vi "gsp_simulator_write_response.vi"(4 "error in (no error)":errorcluster, 5 "Parameters":i32[](array[numeric]), 6 "Motor#":u8, 7 "Command#":u16) -> (0 "error out":errorcluster)   [LabVIEW 2015]
uses:
  gsp_simulator_global.vi
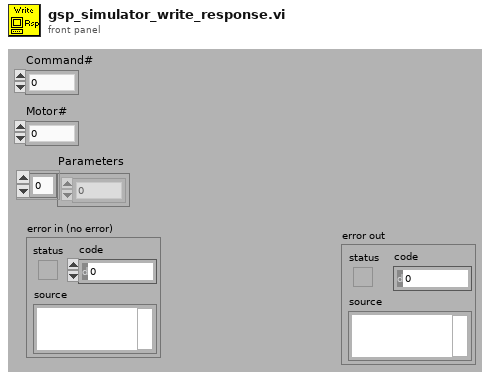
[diagram p1: front panel]
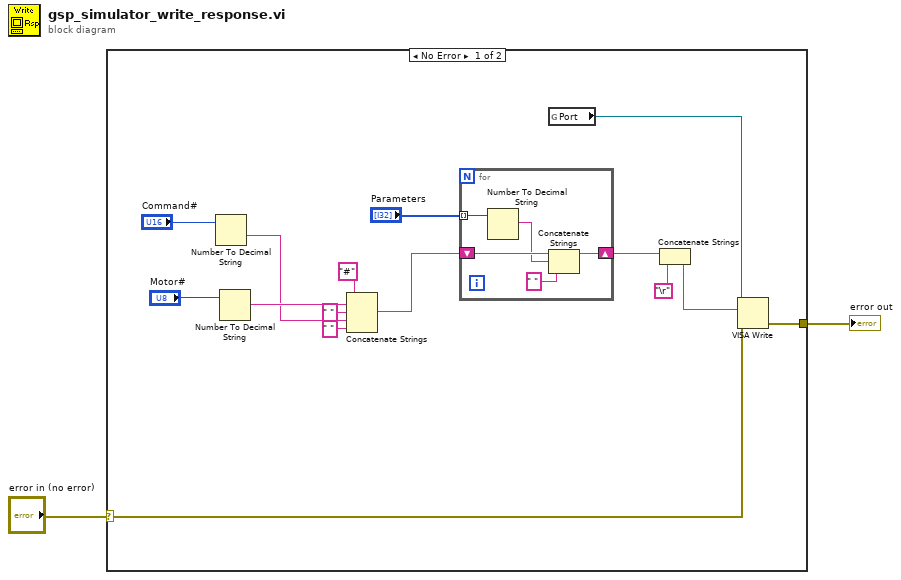
[diagram p0: block diagram]
diagram:
  n1 = case shown="No Error" "error in (no error)" {
    selector: "error in (no error)" -> [w3 w23]
    tunnel: [w16 w23] -> w2
    frame No Error {
      n2 = Number To Decimal String(number="Command#") -> (decimal integer string=w10:string)  [unwired: 1 in]
      n3 = Number To Decimal String(number="Motor#") -> (decimal integer string=w13:string)  [unwired: 1 in]
      n4 = Concatenate Strings("#", w13, " " ("string"), w10, " " ("string")) -> (w8:string)
      n5 = for {
        tunnel: "Parameters" -> [w22] mode=indexing
        shift-right: [w18] -> w7
        shift-left: w8 -> [w21]
        n6 = Number To Decimal String(number=w22) -> (decimal integer string=w19:string)  [unwired: 1 in]
        n7 = Concatenate Strings(w21, w19, " " ("string")) -> (w18:string)
      }
      n8 = global read "gsp_simulator_global.vi" "Port"() -> (w17:refnum<visa-resource-name>)
      n9 = Concatenate Strings(w7, "\r") -> (w5:string)
      n10 = VISA Write(VISA resource name=w17, write buffer=w5, error in (no error)=w3) -> (error out=w16:errorcluster)  [unwired: 2 out]
    }
    frame Error {
    }
  }
  "error out" <- w2
